vi "Read Length.vi"(8 "error in (no error)":errorcluster, 11 "Spk Cycle MSG in":refnum<class "Spk Cycle MSG.lvclass">) -> (0 "error out":errorcluster, 2 "Length":i16, 3 "Spk Cycle MSG out":refnum<class "Spk Cycle MSG.lvclass">)   [LabVIEW 2014, in "ePAS Library.lvlib" / "Spk Cycle MSG.lvclass"]
uses:
  Spk Cycle MSG.lvclass
  Spk Cycle MSG.lvclass/Spk Cycle MSG.ctl
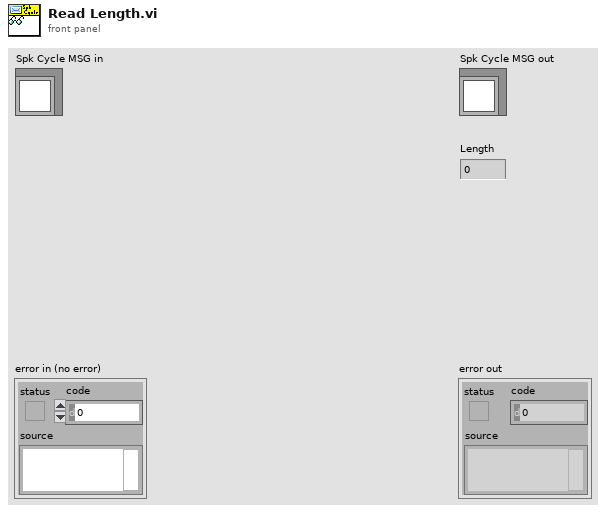
[diagram p1: front panel]
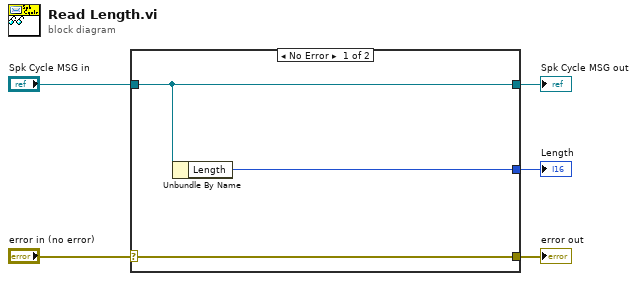
[diagram p0: block diagram]
diagram:
  n1 = case shown="No Error" "error in (no error)" {
    selector: "error in (no error)" -> [w8 w9]
    tunnel: [w8 w9] -> w4
    tunnel: [w7 w10] -> w2
    tunnel: "Spk Cycle MSG in" -> [w7 w10]
    tunnel: [w6 _] -> w1
    frame No Error {
      n2 = Unbundle By Name(w7) -> ("Length"=w6:i16)
    }
    frame Error {
    }
  }
  "error out" <- w4
  "Spk Cycle MSG out" <- w2
  "Length" <- w1
